vi "Set Temperature.vi"(8 "error in (no error)":errorcluster, 11 "Simulated_CCD_Camera in":refnum<class "Simulated_CCD_Camera.lvclass">) -> (0 "error out":errorcluster, 3 "Simulated_CCD_Camera out":refnum<class "Simulated_CCD_Camera.lvclass">)   [LabVIEW 2018, in "Simulated_CCD_Camera.lvclass"]
uses:
  Simulated_CCD_Camera.lvclass
  Simulated_CCD_Camera.lvclass/Simulated_CCD_Camera.ctl
  Interface/Interface.lvclass/Interface.ctl
  Interface/Interface.lvclass
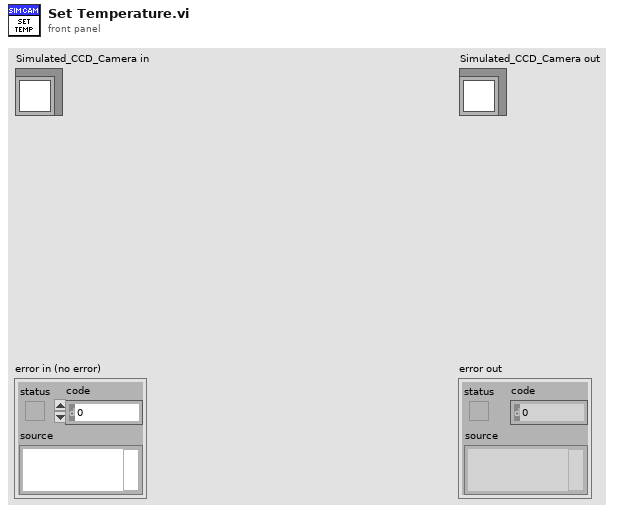
[diagram p1: front panel]
types:
  T1 = cluster{"COOLER_POWER_STATUS":u16, "TEMP":i32, "EXPTIME":dbl, "#FRAMES":u32, "#CUBES":u32}
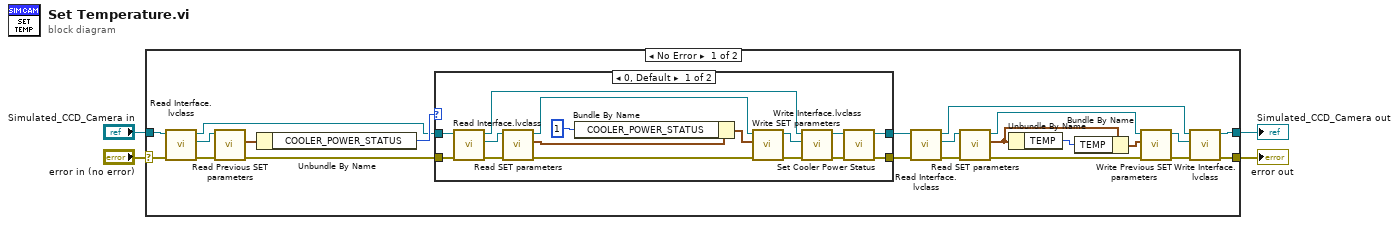
[diagram p0: block diagram]
diagram:
  n1 = case shown="No Error" "error in (no error)" {
    selector: "error in (no error)" -> [w23 w46]
    tunnel: [w7 w46] -> w3
    tunnel: [w8 w45] -> w1
    tunnel: "Simulated_CCD_Camera in" -> [w24 w45]
    frame No Error {
      n2 = call "Read Interface.lvclass.vi"("error in (no error)"=w23, "Simulated_CCD_Camera in"=w24) -> ("error out"=w20:errorcluster, "Interface.lvclass"=w21:refnum<class "Interface.lvclass">, "Simulated_CCD_Camera out"=w25:refnum<class "Simulated_CCD_Camera.lvclass">)  [unwired: 7 in]
      n3 = call "Read Previous SET parameters.vi"("error in (no error)"=w20, "Interface in"=w21) -> ("error out"=w19:errorcluster, "Previous SET parameters"=w22:T1)  [unwired: 7 in, 1 out]
      n4 = Unbundle By Name(w22) -> ("COOLER_POWER_STATUS"=w26:u16)
      n5 = case shown="0, Default" w26 {
        tunnel: w19 -> [w39 w44]
        tunnel: [w28 w44] -> w17
        tunnel: w25 -> [w40 w43]
        tunnel: [w29 w43] -> w18
        frame 0, Default {
          n6 = call "Read Interface.lvclass.vi"("error in (no error)"=w39, "Simulated_CCD_Camera in"=w40) -> ("error out"=w36:errorcluster, "Interface.lvclass"=w35:refnum<class "Interface.lvclass">, "Simulated_CCD_Camera out"=w41:refnum<class "Simulated_CCD_Camera.lvclass">)  [unwired: 7 in]
          n7 = call "Read SET parameters.vi"("error in (no error)"=w36, "Interface in"=w35) -> ("error out"=w31:errorcluster, "SET parameters"=w34:T1, "Interface out"=w32:refnum<class "Interface.lvclass">)  [unwired: 7 in]
          n8 = Bundle By Name(cluster=w34, "COOLER_POWER_STATUS"=u16 1) -> (w33:T1)
          n9 = call "Write SET parameters.vi"("error in (no error)"=w31, "SET parameters"=w33, "Interface in"=w32) -> ("error out"=w37:errorcluster, "Interface out"=w38:refnum<class "Interface.lvclass">)  [unwired: 7 in]
          n10 = call "Write Interface.lvclass.vi"("error in (no error)"=w37, "Interface.lvclass"=w38, "Simulated_CCD_Camera in"=w41) -> ("error out"=w27:errorcluster, "Simulated_CCD_Camera out"=w30:refnum<class "Simulated_CCD_Camera.lvclass">)  [unwired: 7 in]
          n11 = call-dynamic "Set Cooler Power Status.vi"("error in (no error)"=w27, "Simulated_CCD_Camera in"=w30) -> ("error out"=w28:errorcluster, "Simulated_CCD_Camera out"=w29:refnum<class "Simulated_CCD_Camera.lvclass">)  [unwired: 8 in]
        }
        frame 1 {
        }
      }
      n12 = call "Read Interface.lvclass.vi"("error in (no error)"=w17, "Simulated_CCD_Camera in"=w18) -> ("error out"=w15:errorcluster, "Interface.lvclass"=w16:refnum<class "Interface.lvclass">, "Simulated_CCD_Camera out"=w9:refnum<class "Simulated_CCD_Camera.lvclass">)  [unwired: 7 in]
      n13 = call "Read SET parameters.vi"("error in (no error)"=w15, "Interface in"=w16) -> ("error out"=w12:errorcluster, "SET parameters"=w6:T1, "Interface out"=w13:refnum<class "Interface.lvclass">)  [unwired: 7 in]
      n14 = Unbundle By Name(w6) -> ("TEMP"=w5:i32)
      n15 = Bundle By Name(cluster=w6, "TEMP"=w5) -> (w14:T1)
      n16 = call "Write Previous SET parameters.vi"("error in (no error)"=w12, "Previous SET parameters"=w14, "Interface in"=w13) -> ("error out"=w11:errorcluster, "Interface out"=w10:refnum<class "Interface.lvclass">)  [unwired: 7 in]
      n17 = call "Write Interface.lvclass.vi"("error in (no error)"=w11, "Interface.lvclass"=w10, "Simulated_CCD_Camera in"=w9) -> ("error out"=w7:errorcluster, "Simulated_CCD_Camera out"=w8:refnum<class "Simulated_CCD_Camera.lvclass">)  [unwired: 7 in]
    }
    frame Error {
    }
  }
  "error out" <- w3
  "Simulated_CCD_Camera out" <- w1
